vi "young_tipcounter.vi"(0 "Poll Response (TB Count)":i32, 3 "TB In":i32, 5 "Tips In":i32, 7 "Current Time":timestamp) -> (14 "Cumulative Tip Count":dbl, 15 "Rain Rate":dbl, 16 "Cumulative Rain Fall":dbl, 17 "TB Out":i32, 19 "Tips Out":i32)   [LabVIEW 2018]
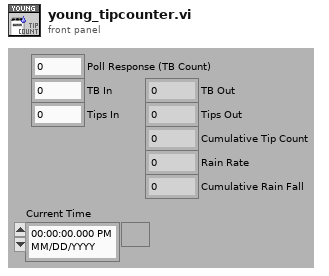
[diagram p1: front panel]
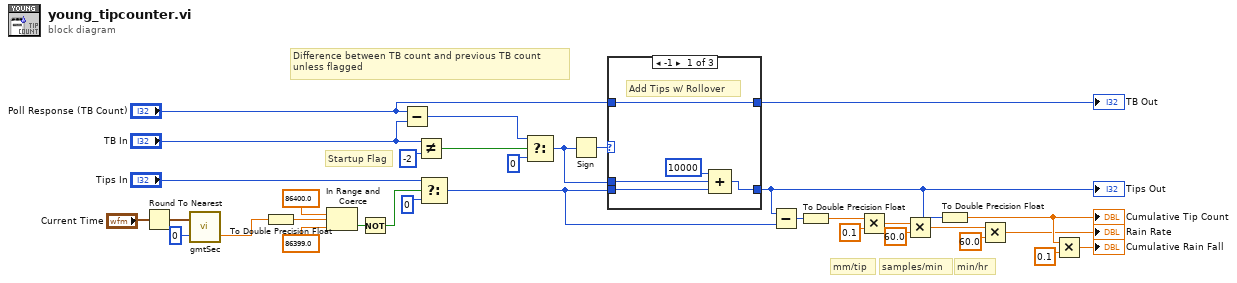
[diagram p0: block diagram]
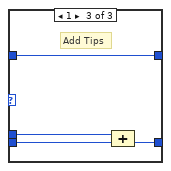
[diagram p3: hidden frame]
diagram:
  # "Difference between TB count and previous TB count\nunless flagged"
  # "Startup Flag"
  # "min/hr"
  # "samples/min"
  # "mm/tip"
  n1 = Round To Nearest(number="Current Time") -> (nearest integer value=w7:timestamp)
  n2 = call "gmtSec.vi"("Timezone Offset (Hrs)"=0, "Timestamp"=w7) -> ("Fractional Sec Since 12AM GMT"=w5:dbl)  [unwired: 1 out]
  n3 = To Double Precision Float(number=w5) -> (double precision float=w25:dbl)
  n4 = In Range and Coerce(upper limit=86400.0, x=w25, lower limit=86399.0) -> (In Range?=w23:bool)  [unwired: 1 out]
  n5 = Not(x=w23) -> (.not. x?=w24:bool)
  n6 = Subtract(x="Poll Response (TB Count)", y="TB In") -> (x-y=w13:i32)
  n7 = Not Equal?(x="TB In", y=-2) -> (x != y?=w14:bool)
  n8 = Select(t="Tips In", s=w24, f=0) -> (s? t:f=w9:i32)
  n9 = Select(t=w13, s=w14, f=0) -> (s? t:f=w12:i32)
  n10 = Sign(1:w12) -> (0:w17:i32)
  n11 = case shown="-1" w17 {
    tunnel: [w34 w39 w41] -> w10
    tunnel: w12 -> [w36 _ w43]
    tunnel: [w38 w40 w44] -> w18
    tunnel: "Poll Response (TB Count)" -> [w38 w40 w44]
    tunnel: w9 -> [w37 w39 w42]
    frame -1 {
      # "Add Tips w/ Rollover"
      n12 = Compound Arithmetic op=ADD(10000 ("value"), w36, w37) -> (w34:i32)
    }
    frame 0, Default {
      # "No Tips"
    }
    frame 1 {
      # "Add Tips"
      n13 = Compound Arithmetic op=ADD(w43, w42) -> (w41:i32)
    }
  }
  "Tips Out" <- w10
  "TB Out" <- w18
  n14 = Subtract(x=w10, y=w9) -> (x-y=w8:i32)
  n15 = To Double Precision Float(number=w8) -> (double precision float=w30:dbl)
  n16 = Multiply(x=w30, y=0.1) -> (x*y=w33:dbl)
  n17 = Multiply(x=w33, y=60.0) -> (x*y=w3:dbl)
  n18 = To Double Precision Float(number=w10) -> (double precision float=w28:dbl)
  "Cumulative Tip Count" <- w28
  n19 = Multiply(x=w3, y=60.0) -> (x*y=→"Rain Rate":dbl)
  n20 = Multiply(x=w28, y=0.1) -> (x*y=→"Cumulative Rain Fall":dbl)
